vi "vo.vi"(11 "Platter in":T1 format="%032b") -> (4 "V":T1 format="%032b", 6 "O":i32)   [LabVIEW 2020]
uses:
  Platter.ctl
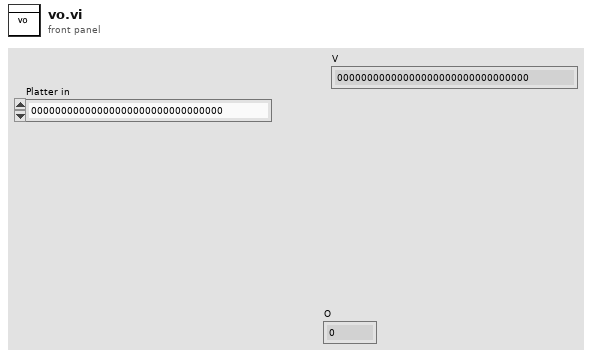
[diagram p1: front panel]
types:
  T1 = typedef "Platter.ctl" = u32
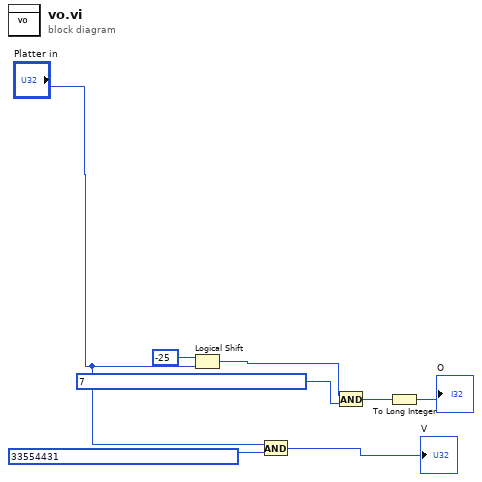
[diagram p0: block diagram]
diagram:
  n1 = Logical Shift(y=i16 -25, x="Platter in") -> (x << y=w3:T1)
  n2 = And(x="Platter in", y=T1 33554431) -> (x .and. y?=→"V":T1)
  n3 = And(x=w3, y=T1 7) -> (x .and. y?=w2:T1)
  n4 = To Long Integer(number=w2) -> (32bit integer=→"O":i32)
